vi "Set Stop Trigger (Duration).vi"(8 "error in (no error)":errorcluster, 10 "Duration":dbl, 11 "Data Logging Specification Ref in":T1) -> (0 "error out":errorcluster, 3 "Data Logging Specification Ref out":T1)   [LabVIEW 2020, in "NI_VS Data Logging API.lvlib"]
doc: "Specifies a trigger condition on which to stop logging data. You also can specify whether to continue logging channel data for a set period of time after the trigger condition occurs.\n\nYou must manually select the polymorphic instance to use."
uses:
  <vilib>/NI VeriStand/Execution/DataLogging/NI_VS Data Logging API.lvlib
  <vilib>/NI VeriStand/Execution/DataLogging/DataLoggingSpecification Ref.ctl
  NationalInstruments.VeriStand.ClientAPI
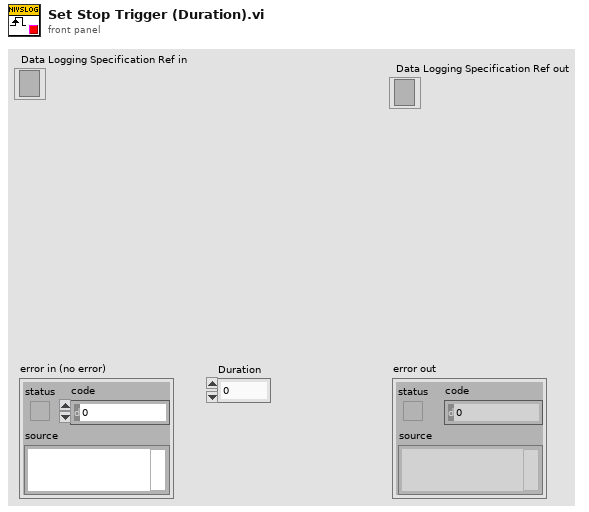
[diagram p1: front panel]
types:
  T1 = typedef "NI_VS Data Logging API.lvlib/DataLoggingSpecification Ref.ctl" = refnum<k24>
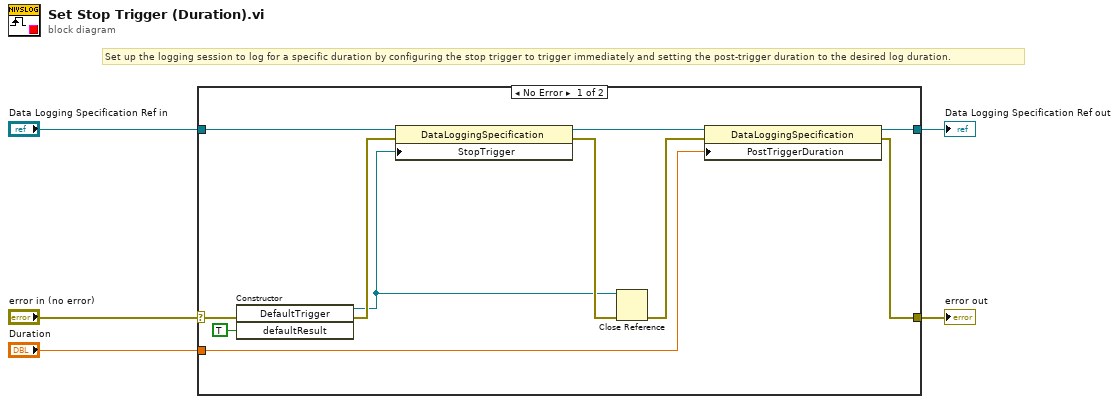
[diagram p0: block diagram]
diagram:
  # "Set up the logging session to log for a specific duration by configuring the stop trigger to trigger immediately and setting the post-trigger duration to the desired log duration."
  n1 = case shown="No Error" "error in (no error)" {
    selector: "error in (no error)" -> [w8 w18]
    tunnel: "Data Logging Specification Ref in" -> [w14 w17]
    tunnel: "Duration" -> [w13 _]
    tunnel: [w10 w17] -> w3
    tunnel: [w9 w18] -> w2
    frame No Error {
      n2 = constructor class="DefaultTrigger"(error in=w8, "defaultResult"=TRUE) -> (reference out=w7:refnum<k24>, error out=w16:errorcluster)  [unwired: 2 in, 2 out]
      n3 = property class="DataLoggingSpecification"(reference=w14, error in=w16, "StopTrigger"=w7) -> (reference out=w12:T1, error out=w15:errorcluster)
      n4 = Close Reference(reference=w7, error in (no error)=w15) -> (error out=w11:errorcluster)
      n5 = property class="DataLoggingSpecification"(reference=w12, error in=w11, "PostTriggerDuration"=w13) -> (reference out=w10:T1, error out=w9:errorcluster)
    }
    frame Error {
    }
  }
  "error out" <- w2
  "Data Logging Specification Ref out" <- w3
